vi "DIGITIZER_CHANNEL_SELECTION.vi"(9 "Channel Name":string) -> (0 "DIGITIZER 2 CHANNELS":string, 1 "DIGITIZER 2 USED?":bool, 2 "DIGITIZER 1 CHANNELS":string, 3 "DIGITIZER 1 USED?":bool, 4 "PARTIAL DIGITIZER PARAMETERS CLUSTER":T1)   [LabVIEW 2010]
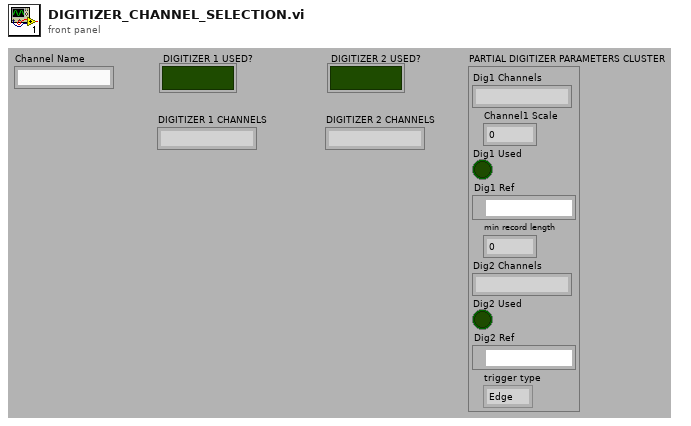
[diagram p1: front panel]
types:
  T1 = cluster{"Dig1 Channels":string, "Channel1 Scale":dbl, "Dig1 Used":bool, "Dig1 Ref":refnum<k15>, "min record length":i32, "Dig2 Channels":string, "Dig2 Used":bool, "Dig2 Ref":refnum<k15>, "trigger type":enum16{"Edge", "Digital", "Immediate"}}
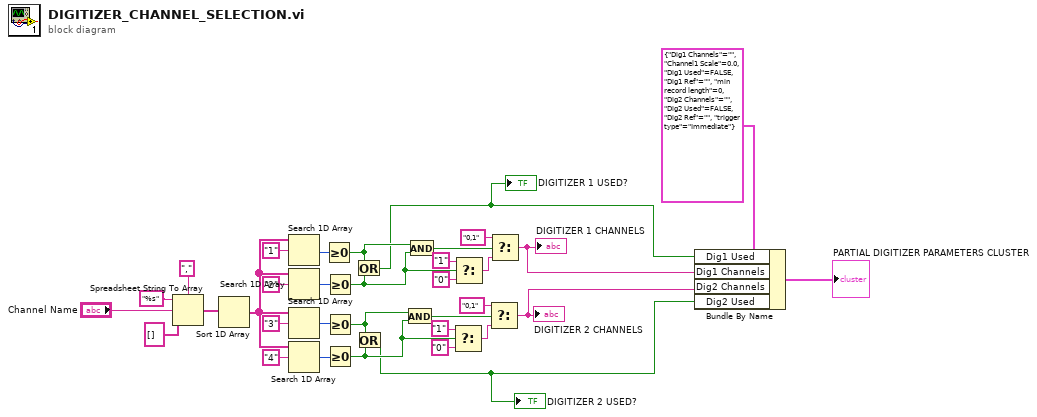
[diagram p0: block diagram]
diagram:
  n1 = Spreadsheet String To Array(delimiter (Tab)=",", format string="%s", spreadsheet string="Channel Name", array type (2D Dbl)=string[] []) -> (array=w10:string[])
  n2 = Sort 1D Array(array=w10) -> (sorted array=w11:string[])
  n3 = Search 1D Array(1D array=w11, element="1") -> (index of element=w16:i32)  [unwired: 1 in]
  n4 = Search 1D Array(1D array=w11, element="2") -> (index of element=w19:i32)  [unwired: 1 in]
  n5 = Search 1D Array(1D array=w11, element="3") -> (index of element=w18:i32)  [unwired: 1 in]
  n6 = Search 1D Array(1D array=w11, element="4") -> (index of element=w17:i32)  [unwired: 1 in]
  n7 = Greater Or Equal To 0?(x=w16) -> (x >= 0?=w20:bool)
  n8 = Greater Or Equal To 0?(x=w19) -> (x >= 0?=w24:bool)
  n9 = Greater Or Equal To 0?(x=w18) -> (x >= 0?=w21:bool)
  n10 = Greater Or Equal To 0?(x=w17) -> (x >= 0?=w33:bool)
  n11 = Or(x=w20, y=w24) -> (x .or. y?=w2:bool)
  "DIGITIZER 1 USED?" <- w2
  n12 = Or(x=w21, y=w33) -> (x .or. y?=w5:bool)
  "DIGITIZER 2 USED?" <- w5
  n13 = And(x=w21, y=w33) -> (x .and. y?=w32:bool)
  n14 = And(x=w20, y=w24) -> (x .and. y?=w22:bool)
  n15 = Select(t="1", s=w33, f="0") -> (s? t:f=w30:string)
  n16 = Select(t="1", s=w24, f="0") -> (s? t:f=w26:string)
  n17 = Select(t="0,1", s=w32, f=w30) -> (s? t:f=w6:string)
  "DIGITIZER 2 CHANNELS" <- w6
  n18 = Select(t="0,1", s=w22, f=w26) -> (s? t:f=w1:string)
  "DIGITIZER 1 CHANNELS" <- w1
  n19 = Bundle By Name(cluster=T1 {"Dig1 Channels"="", "Channel1 Scale"=0.0, "Dig1 Used"=FALSE, "Dig1 Ref"="", "min record length"=0, "Dig2 Channels"="", "Dig2 Used"=FALSE, "Dig2 Ref"="", "trigger type"=enum."Immediate"}, "Dig1 Used"=w2, "Dig1 Channels"=w1, "Dig2 Channels"=w6, "Dig2 Used"=w5) -> (→"PARTIAL DIGITIZER PARAMETERS CLUSTER":T1)
